vi "Check and Log Plugin Timeout Error.vi"(6 "-1014 timeout (ms)":u32=10000, 7 "Plugin Subpanel Events":T1, 8 "New Error":errorcluster, 10 "Previous Error":errorcluster, 11 "CIF_UI in":refnum<class "CIF_UI.lvclass">) -> (0 "error out":errorcluster, 3 "CIF_UI out":refnum<class "CIF_UI.lvclass">)   [LabVIEW 2021, in "CIF_UI.lvclass"]
doc: "This error management and logging VI is intended to run in the timeout case of the event structure in plugin UI loops. It will manage the registration of new local errors by checking if a previous, uncleared, error exists.\n\nIt will also mute specific errors and check for use cases where the plugin should shutdown automatically."
uses:
  CIF_UI.lvclass
  Typedef/Plugin Subpanel Events.ctl
  CIF_UI.lvclass/CIF_UI.ctl
  Utilities/Get Human Readable Error.vi
  <vilib>/CIF Foundation/CIF Utilities/Errors/Append Error Location.vi
  <vilib>/CIF Foundation/CIF Utilities/Errors/Human Readable Error Message.vi
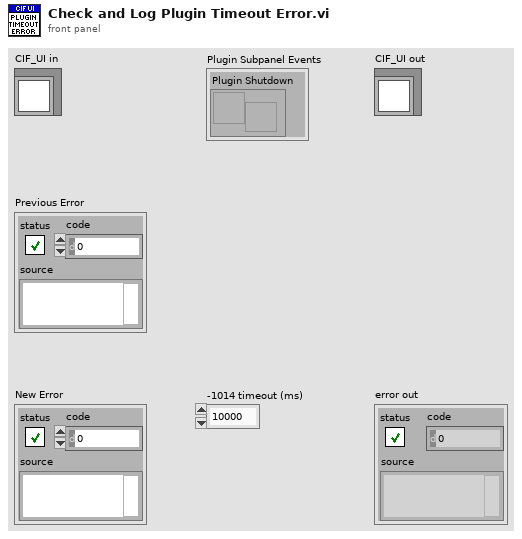
[diagram p1: front panel]
types:
  T1 = typedef "CIF_UI.lvclass/Plugin Subpanel Events.ctl" = cluster{"Plugin Shutdown":refnum<user-event>}
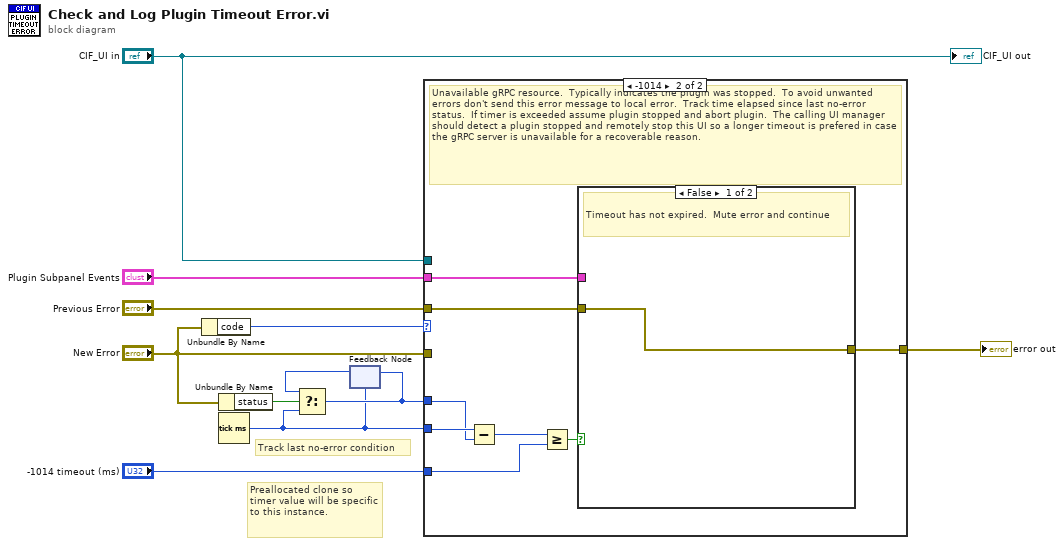
[diagram p0: block diagram]
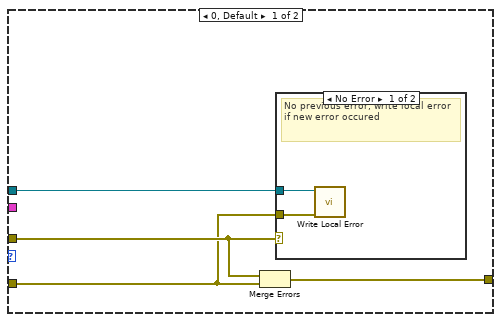
[diagram p2: hidden frame]
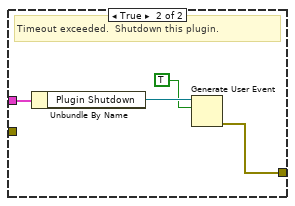
[diagram p4: hidden frame]
diagram:
  # "Preallocated clone so timer value will be specific to this instance."
  # "Track last no-error condition"
  n1 = Unbundle By Name("New Error") -> ("code"=w8:i32)
  n2 = Unbundle By Name("New Error") -> ("status"=w6:bool)
  n3 = Tick Count (ms)() -> (millisecond timer value=w3:u32)
  n4 = feedback #1(w3) -> (w5:u32)
  n5 = Select(t=w5, s=w6, f=w3) -> (s? t:f=w4:u32)
  n6 = feedback-in #1(w4) -> ()
  n7 = case shown="-1014" w8 {
    tunnel: "Previous Error" -> [w15 w18]
    tunnel: [w14 w19] -> w10
    tunnel: "CIF_UI in" -> [w13 _]
    tunnel: "New Error" -> [w12 _]
    tunnel: w4 -> [_ w24]
    tunnel: w3 -> [_ w25]
    tunnel: "-1014 timeout (ms)" -> [_ w22]
    tunnel: "Plugin Subpanel Events" -> [_ w20]
    frame 0, Default {
      n8 = Merge Errors(w15, w12) -> (w14:errorcluster)
      n9 = case shown="No Error" w15 {
        tunnel: w13 -> [w17 _]
        tunnel: w12 -> [w16 _]
        frame No Error {
          # "No previous error, write local error if new error occured"
          n10 = call "Write Local Error.vi"("error in (no error)"=w16, "CIF_UI in"=w17) -> ()  [unwired: 9 in, 1 out]
        }
        frame Error {
        }
      }
    }
    frame -1014 {
      # "Unavailable gRPC resource.  Typically indicates the plugin was stopped.  To avoid unwanted errors don't send this error message to local error.  Track time elapsed since last no-error status.  If timer is exceeded assume plugin stopped and abort plugin.  The calling UI manager should detect a plugin stopped and remotely stop this UI so a longer timeout is prefered in case the gRPC server is unavailable for a recoverable reason."
      n11 = Subtract(x=w25, y=w24) -> (x-y=w23:u32)
      n12 = Greater Or Equal?(x=w23, y=w22) -> (x >= y?=w21:bool)
      n13 = case shown="False" w21 {
        tunnel: w20 -> [_ w30]
        tunnel: [w26 w27] -> w19
        tunnel: w18 -> [w26 _]
        frame False {
          # "Timeout has not expired.  Mute error and continue"
        }
        frame True {
          # "Timeout exceeded.  Shutdown this plugin."
          n14 = Unbundle By Name(w30) -> ("Plugin Shutdown"=w29:refnum<user-event>)
          n15 = Generate User Event(user event=w29, event data cluster=TRUE ("event data")) -> (error out=w27:errorcluster)  [unwired: 2 in, 1 out]
        }
      }
    }
  }
  "error out" <- w10
  "CIF_UI out" <- "CIF_UI in"
